vi "Configure Stream.vi"(0 "niUsrpRio Session":T1={"Global Settings Register Bus"=refnum, "Radio 0 Settings Register Bus"=refnum, "Rx NI-USRP session"="", "Tx NI-USRP session"="", "FPGA Interface"=refnum, "RIO Interface Number"=0, "EEPROM Header"={"Checksum"=0, "Product Code"=0, "Hardware Current Version"=0, "Hardware Oldest Compatible Version"=0, "EEPROM Map Current Version"=0, "EEPROM Map Oldest Compatible Version"=0, "User Password"="", "Pointer to Factory Header"=0, "Pointer to User Header"=0, "Recommended Interval"=0, "Number of Reserved Bytes"=9, "Number of Daughterboards"=0, "Daughterboard IDs"=[], "Daughterboard Serial Numbers"=[]}, "Device Data Header"={"Checksum"=0, "Number of Channels"=0, "Number of Gain Settings"=[], "Pointer to Characterization Data"=[], "Number of Reserved Bytes"=27, "Number of Frequencies"=[]}, "EEPROM Characterization Header"={"Checksum"=0, "Date"=timestamp(0 s since 1904-01-01), "Temperature"=0.0, "Misc. Info"="", "Pointer to Device Data Header"=0, "Number of Reserved Bytes"=28}, "Characterization Data"=[], "Characterization Data Valid?"=FALSE, "Radio 1 Settings Register Bus"=refnum, "Radio Settings Bus Semaphore"=refnum} {"Characterization Data"."Frequencies [Hz]" format="%#_6p"; "EEPROM Characterization Header"."Pointer to Device Data Header" format="%x"; "EEPROM Characterization Header"."Checksum" format="%x"; "Device Data Header"."Pointer to Characterization Data" format="%x"; "Device Data Header"."Checksum" format="%x"; "EEPROM Header"."Pointer to User Header" format="%x"; "EEPROM Header"."Pointer to Factory Header" format="%x"; "EEPROM Header"."Product Code" format="%x"; "EEPROM Header"."Checksum" format="%x"}, 1 "scope":string(combo)="rx", 5 "host FIFO depth":u32=1000000 format="%.0p", 7 "number of samples is finite":bool caption="Number of Samples is Finite", 9 "number of samples":u32=8192 caption="Number of Samples", 11 "error in":errorcluster) -> (4 "niUsrpRio Session (out)":T1={"Global Settings Register Bus"=refnum, "Radio 0 Settings Register Bus"=refnum, "Rx NI-USRP session"="", "Tx NI-USRP session"="", "FPGA Interface"=refnum, "RIO Interface Number"=0, "EEPROM Header"={"Checksum"=0, "Product Code"=0, "Hardware Current Version"=0, "Hardware Oldest Compatible Version"=0, "EEPROM Map Current Version"=0, "EEPROM Map Oldest Compatible Version"=0, "User Password"="", "Pointer to Factory Header"=0, "Pointer to User Header"=0, "Recommended Interval"=0, "Number of Reserved Bytes"=9, "Number of Daughterboards"=0, "Daughterboard IDs"=[], "Daughterboard Serial Numbers"=[]}, "Device Data Header"={"Checksum"=0, "Number of Channels"=0, "Number of Gain Settings"=[], "Pointer to Characterization Data"=[], "Number of Reserved Bytes"=27, "Number of Frequencies"=[]}, "EEPROM Characterization Header"={"Checksum"=0, "Date"=timestamp(0 s since 1904-01-01), "Temperature"=0.0, "Misc. Info"="", "Pointer to Device Data Header"=0, "Number of Reserved Bytes"=28}, "Characterization Data"=[], "Characterization Data Valid?"=FALSE, "Radio 1 Settings Register Bus"=refnum, "Radio Settings Bus Semaphore"=refnum} {"Characterization Data"."Frequencies [Hz]" format="%#_6p"; "EEPROM Characterization Header"."Pointer to Device Data Header" format="%x"; "EEPROM Characterization Header"."Checksum" format="%x"; "Device Data Header"."Pointer to Characterization Data" format="%x"; "Device Data Header"."Checksum" format="%x"; "EEPROM Header"."Pointer to User Header" format="%x"; "EEPROM Header"."Pointer to Factory Header" format="%x"; "EEPROM Header"."Product Code" format="%x"; "EEPROM Header"."Checksum" format="%x"}, 15 "error out":errorcluster)   [LabVIEW 2013]
doc: "Configures the stream. This includes configuring the DMA FIFO and the Rx/Tx stream size (in samples).\n\n<B>Input Parameters</B>\n\n<B>niUsrpRio Session</B> is the object created by the Open VI and used as the session handle for the USRP RIO design library.\n\n<B>scope</B> is the channel to configure the stream for. The options are \"rx/RF 0\", \"rx/RF 1\", \"tx/RF 0\", and \"tx/RF 1\".\n\n<B>host FIFO depth</B> is the number of samples of buffering to request on the host. This value is optional and defaults to eight times the 'number of samples'.\n\n<B>number of samples is finite</B> is used to flag whether this is a continuous acquisition/generation or a finite acquisition/generation.\n\n<B>number of samples</B> to acquire/generate.\n\n<B>error in</B> describes error conditions that occur before this node runs. This input provides standard 'error in' functionality.\n\n<B>Output Parameters</B>\n\n<B>niUsrpRio Session (out)</B> is the niUsrpRio session used in all subsequent USRP RIO design library host VIs.\n\n<B>error out</B> contains error information. This output provides standard 'error out' functionality."
uses:
  <instrlib>/niUsrpRio/Config/v1/Host/Public/niUsrpRio Session.ctl
  <instrlib>/_niInstr/Register Bus/v0/Host/Public/Register Bus Session.ctl
  <instrlib>/_niInstr/Register Bus/v0/Host/Private/Session Data.ctl
  <instrlib>/niUsrpRio/Config/v1/Host/Public/EEPROM Header.ctl
  <instrlib>/niUsrpRio/Config/v1/Host/Public/EEPROM Device Data Header.ctl
  <instrlib>/niUsrpRio/Config/v1/Host/Public/EEPROM Characterization Header.ctl
  <instrlib>/niUsrpRio/Config/v1/Host/Public/Characterization Data.ctl
  <instrlib>/niUsrpRio/Config/v1/Host/Public/IQ Imbalance.ctl
  Tx FPGA VI Reference.ctl
  Rx FPGA VI Reference.ctl
  <vilib>/rvi/interface/common/niFpgaWaitOnOcc.vi
  <vilib>/Utility/error.llb/Error Cluster From Error Code.vi
  <vilib>/rvi/errors/niLvFpgaAdjustHostInterfaceError.vi
  <vilib>/ErrorRing/Error Ring.xnode
  <vilib>/rvi/interface/nirviReadWriteControl/nirviReadWriteControl.xnode
  <vilib>/rvi/interface/nirviMethod/nirviMethod.xnode
  <vilib>/rvi/errors/niLvFpgaMergeErrorWithErrorCode.vi
  <vilib>/rvi/interface/Simulation/niFpgaSimulationCallBeginRW.vi
  NiFpgaLv.dll
  <vilib>/FPGAPlugInAG/Dynamic/niLvFpga_StartFifo_Dynamic.vi
  <vilib>/FPGAPlugInAG/Dynamic/niLvFpga_StopFifo_Dynamic.vi
  <vilib>/FPGAPlugInAG/Dynamic/niLvFpga_ConfigureFifo_Dynamic.vi
  <instrlib>/niUsrpRio/Config/v1/Host/niUsrpRio Config v1 Host.lvlib
  <instrlib>/_niInstr/Register Bus/v0/Host/niInstr Register Bus v0 Host.lvlib
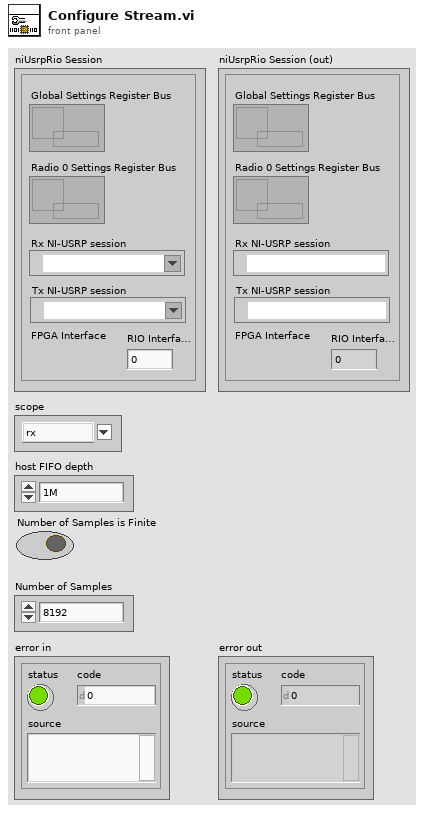
[diagram p1: front panel]
types:
  T1 = typedef "niUsrpRio Config v1 Host.lvlib/niUsrpRio Session.ctl" = cluster{"Global Settings Register Bus":T2, "Radio 0 Settings Register Bus":T2, "Rx NI-USRP session":refnum<k15>, "Tx NI-USRP session":refnum<k15>, "FPGA Interface":refnum<k20>, "RIO Interface Number":u32, "EEPROM Header":T3, "Device Data Header":T4, "EEPROM Characterization Header":T5, "Characterization Data":T6[], "Characterization Data Valid?":bool, "Radio 1 Settings Register Bus":T2, "Radio Settings Bus Semaphore":T8}
  T2 = typedef "niInstr Register Bus v0 Host.lvlib/Register Bus Session.ctl" = refnum<queue>
  T3 = typedef "niUsrpRio Config v1 Host.lvlib/EEPROM Header.ctl" = cluster{"Checksum":u32, "Product Code":u16, "Hardware Current Version":u16, "Hardware Oldest Compatible Version":u16, "EEPROM Map Current Version":u16, "EEPROM Map Oldest Compatible Version":u16, "User Password":string, "Pointer to Factory Header":u32, "Pointer to User Header":u32, "Recommended Interval":u16, "Number of Reserved Bytes":i32, "Number of Daughterboards":u8, "Daughterboard IDs":u16[], "Daughterboard Serial Numbers":string[]}
  T4 = typedef "niUsrpRio Config v1 Host.lvlib/EEPROM Device Data Header.ctl" = cluster{"Checksum":u32, "Number of Channels":u8, "Number of Gain Settings":u16[], "Pointer to Characterization Data":u32[], "Number of Reserved Bytes":i32, "Number of Frequencies":u16[]}
  T5 = typedef "niUsrpRio Config v1 Host.lvlib/EEPROM Characterization Header.ctl" = cluster{"Checksum":u32, "Date":timestamp, "Temperature":sgl, "Misc. Info":string, "Pointer to Device Data Header":u32, "Number of Reserved Bytes":i32}
  T6 = typedef "niUsrpRio Config v1 Host.lvlib/Characterization Data.ctl" = cluster{"Gains[dB]":dbl[], "Frequencies [Hz]":dbl[], "IQ Imbalance Table":T7[], "Measured Gains[dB]":dbl[][]}
  T7 = typedef "niUsrpRio Config v1 Host.lvlib/IQ Imbalance.ctl" = cluster{"Gain Imbalance [linear]":dbl, "Phase Imbalance [radians]":dbl, "Offset":cdb}
  T8 = typedef "Semaphore RefNum" = refnum<k1>
  T9 = typedef "niUsrpRio Config v1 Host.lvlib/Device Subfunction.ctl" = enum16{"rx", "tx"}
  T10 = typedef "niUsrpRio Config v1 Host.lvlib/RF Channel.ctl" = enum16{"0", "1", "All"}
  T11 = typedef "Tx FPGA VI Reference.ctl" = refnum<k20>
  T12 = typedef "Rx FPGA VI Reference.ctl" = refnum<k20>
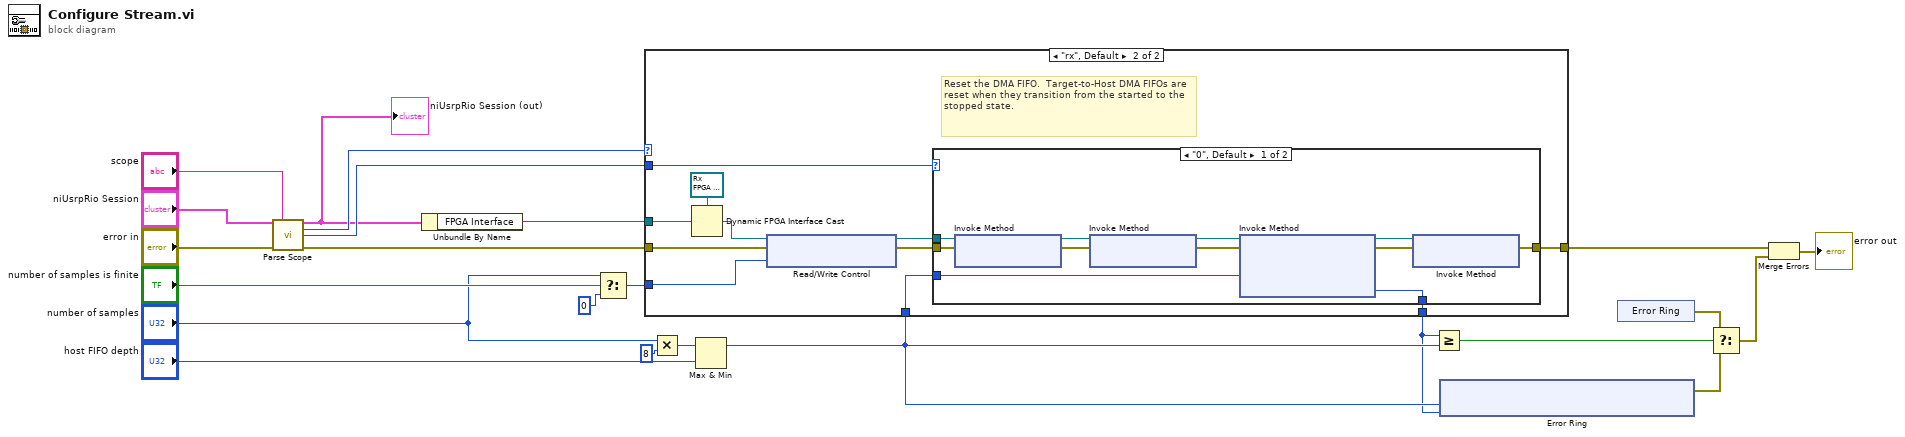
[diagram p0: block diagram]
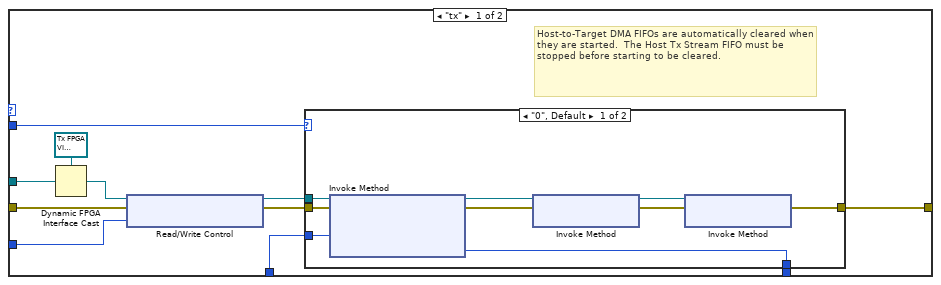
[diagram p2: hidden frame]
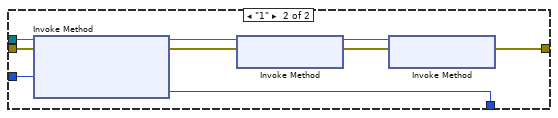
[diagram p3: hidden frame]
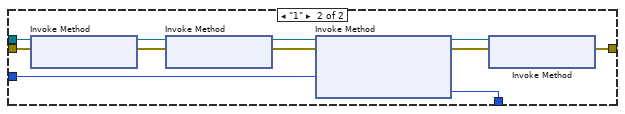
[diagram p4: hidden frame]
diagram:
  n1 = call <instrlib>:"Parse Scope.vi"("niUsrpRio Session"="niUsrpRio Session", "scope"="scope", "Error In"="error in") -> ("niUsrpRio Session (out)"=w6:T1, "Device Subfunction"=w8:T9, "Device Subfunction Channel"=w7:T10, "Error Out"=w4:errorcluster)  [unwired: 4 in, 5 out]
  "niUsrpRio Session (out)" <- w6
  n2 = Unbundle By Name(w6) -> ("FPGA Interface"=w5:refnum<k20>)
  n3 = Select(t="number of samples", s="number of samples is finite", f=u32 0) -> (s? t:f=w17:u32)
  n4 = Multiply(x="number of samples", y=u32 8 ("x")) -> (x*y=w22:u32)
  n5 = Max & Min(x=w22, y="host FIFO depth") -> (max(x,y)=w10:u32)  [unwired: 1 out]
  n6 = case shown="\"rx\", Default" w8 {
    tunnel: w10 -> [w29 w60]
    tunnel: [w33 w62] -> w13
    tunnel: w17 -> [w28 w59]
    tunnel: [w27 w56] -> w9
    tunnel: w5 -> [w26 w55]
    tunnel: w4 -> [w25 w54]
    tunnel: w7 -> [w24 w53]
    frame "tx" {
      # "Host-to-Target DMA FIFOs are automatically cleared when they are started.  The Host Tx Stream FIFO must be stopped before starting to be cleared."
      n7 = Dynamic FPGA Interface Cast(Session In=T11 refnum ("FPGA VI Reference Out"), Type=w26) -> (Session Out=w32:T11)
      n8 = xnode "Read/Write Control"("FPGA VI Reference In"=w32, "error in"=w25, "tx.samples to generate"=w28) -> ("FPGA VI Reference Out"=w30:T11, "error out"=w31:errorcluster)
      n9 = case shown="\"0\", Default" w24 {
        tunnel: [w43 w44] -> w33
        tunnel: w31 -> [w42 w47]
        tunnel: w30 -> [w41 w48]
        tunnel: w29 -> [w36 w46]
        tunnel: [w35 w45] -> w27
        frame "0", Default {
          n10 = xnode "Invoke Method"("FPGA VI Reference In"=w41, "error in"=w42, "Requested Depth"=w36) -> ("FPGA VI Reference Out"=w39:T11, "error out"=w40:errorcluster, "Actual Depth"=w35:u32)
          n11 = xnode "Invoke Method"("FPGA VI Reference In"=w39, "error in"=w40) -> ("FPGA VI Reference Out"=w37:T11, "error out"=w38:errorcluster)
          n12 = xnode "Invoke Method"("FPGA VI Reference In"=w37, "error in"=w38) -> ("error out"=w43:errorcluster)  [unwired: 1 out]
        }
        frame "1" {
          n13 = xnode "Invoke Method"("FPGA VI Reference In"=w48, "error in"=w47, "Requested Depth"=w46) -> ("FPGA VI Reference Out"=w51:T11, "error out"=w52:errorcluster, "Actual Depth"=w45:u32)
          n14 = xnode "Invoke Method"("FPGA VI Reference In"=w51, "error in"=w52) -> ("FPGA VI Reference Out"=w49:T11, "error out"=w50:errorcluster)
          n15 = xnode "Invoke Method"("FPGA VI Reference In"=w49, "error in"=w50) -> ("error out"=w44:errorcluster)  [unwired: 1 out]
        }
      }
    }
    frame "rx", Default {
      # "Reset the DMA FIFO.  Target-to-Host DMA FIFOs are reset when they transition from the started to the stopped state."
      n16 = Dynamic FPGA Interface Cast(Session In=T12 refnum ("Type"), Type=w55) -> (Session Out=w61:T12)
      n17 = xnode "Read/Write Control"("FPGA VI Reference In"=w61, "error in"=w54, "rx.samples to acquire"=w59) -> ("FPGA VI Reference Out"=w57:T12, "error out"=w58:errorcluster)
      n18 = case shown="\"0\", Default" w53 {
        tunnel: [w72 w83] -> w62
        tunnel: w60 -> [w67 w78]
        tunnel: w58 -> [w66 w77]
        tunnel: w57 -> [w65 w76]
        tunnel: [w64 w75] -> w56
        frame "0", Default {
          n19 = xnode "Invoke Method"("FPGA VI Reference In"=w65, "error in"=w66) -> ("FPGA VI Reference Out"=w70:T12, "error out"=w71:errorcluster)
          n20 = xnode "Invoke Method"("FPGA VI Reference In"=w70, "error in"=w71) -> ("FPGA VI Reference Out"=w69:T12, "error out"=w68:errorcluster)
          n21 = xnode "Invoke Method"("FPGA VI Reference In"=w69, "error in"=w68, "Requested Depth"=w67) -> ("FPGA VI Reference Out"=w74:T12, "error out"=w73:errorcluster, "Actual Depth"=w64:u32)
          n22 = xnode "Invoke Method"("FPGA VI Reference In"=w74, "error in"=w73) -> ("error out"=w72:errorcluster)  [unwired: 1 out]
        }
        frame "1" {
          n23 = xnode "Invoke Method"("FPGA VI Reference In"=w76, "error in"=w77) -> ("FPGA VI Reference Out"=w81:T12, "error out"=w82:errorcluster)
          n24 = xnode "Invoke Method"("FPGA VI Reference In"=w81, "error in"=w82) -> ("FPGA VI Reference Out"=w80:T12, "error out"=w79:errorcluster)
          n25 = xnode "Invoke Method"("FPGA VI Reference In"=w80, "error in"=w79, "Requested Depth"=w78) -> ("FPGA VI Reference Out"=w85:T12, "error out"=w84:errorcluster, "Actual Depth"=w75:u32)
          n26 = xnode "Invoke Method"("FPGA VI Reference In"=w85, "error in"=w84) -> ("error out"=w83:errorcluster)  [unwired: 1 out]
        }
      }
    }
  }
  n27 = Greater Or Equal?(x=w9, y=w10) -> (x >= y?=w11:bool)
  n28 = xnode ("Error Ring")("parameter 0"=w10, "parameter 1"=w9) -> ("error out"=w15:errorcluster)
  n29 = xnode ("Error Ring")() -> ("error out"=w14:errorcluster)
  n30 = Select(t=w14, s=w11, f=w15) -> (s? t:f=w16:errorcluster)
  n31 = Merge Errors(w13, w16) -> (→"error out":errorcluster)
